vi "HelpMap.vi"(3 "Control ID":string, 4 "Subitem Help ID":string, 5 "Standard Help ID":string) -> (0 "Control Help Description":string, 1 "Subitem Help Info":T1, 2 "Standard Help Info":T1)   [LabVIEW 2017, in "Get DDT Properties.lvlib" / "Get DDT Properties.xnode"]
uses:
  <vilib>/express/express signal manip/GetorSetDDTAttributes/Get DDT attributes/Get DDT Properties.xnode
panel:
  in  "Control Description":string[](array[string])=["Specifies the index of the signal whose attributes you want to retrieve. The default is 0.", "Specifies the dynamic data that contains the input signal or signals.", "Specifies the index of the signal whose attributes you want to retrieve.", "Describes error conditions that occur before this node runs.", "Returns <B>Signals In</B> unchanged.", "Contains error information. This output provides standard error out functionality.", "Returns the name of the signal.", "Returns the time mode of the signal.", "Returns the timestamp of the signal.", "Returns the start timestamp of the signal.", "Returns the X dimension of the signal.", "Returns the unit of measurement of the signal.", "Specifies whether to return the unit of measurement of the signal.", "Specifies whether to return the X dimension of the signal.", "Specifies whether to return the timestamp of the signal.", "Specifies whether to return the time mode of the signal.", "Specifies whether to return the name of the signal.", "Specifies whether to return the start timestamp of the signal."]
  in  "DNL_Control IDs":string[](array[string])=["Signal Index", "Signals In", "Signal Index", "error in", "Signals Out", "error out", "Signal Name", "Time Mode", "Timestamp", "Start Timestamp", "X Dimension", "Unit", "Unit", "X dimension", "Timestamp", "Time mode", "Signal name", "Start timestamp"]
  in  "Subitem Help Clusters":T2(array[cluster])
  in  "DNL_Subitem Help IDs":string[](array[string])
  in  "Standard Help Clusters":T2(array[cluster])=[{"Description"="Retrieves the attributes of the dynamic data you wire to <B>Signals In</B>.", "Path"=path "<helpdir>/lvexpress.chm", "Tag"="get_ddt_attributes.html"}]
  in  "DNL_Standard Help IDs":string[](array[string])=["Default"]
  # "Description"
  # "Path"
  # "Tag"
  # "Description"
  # "Path"
  # "Tag"
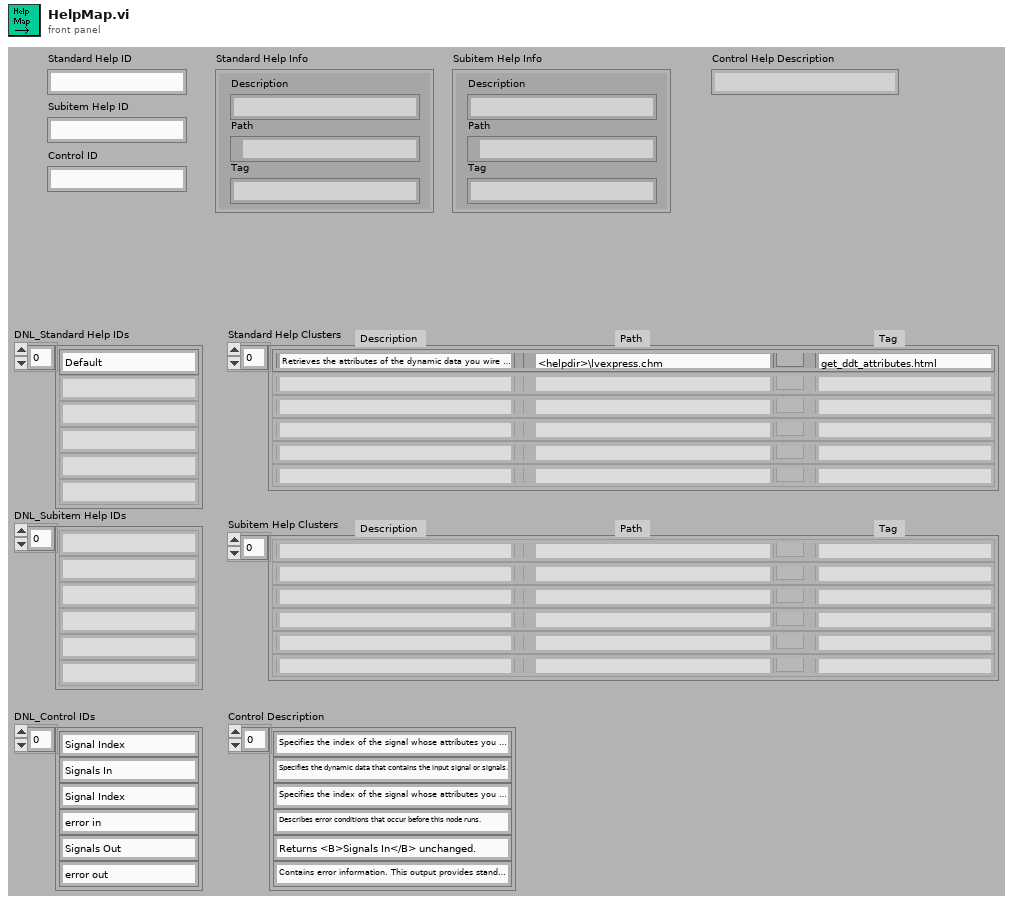
[diagram p1: front panel]
types:
  T1 = cluster{"Description":string, "Path":path, "Tag":string}
  T2 = cluster{"Description":string, "Path":path, "Tag":string}[]
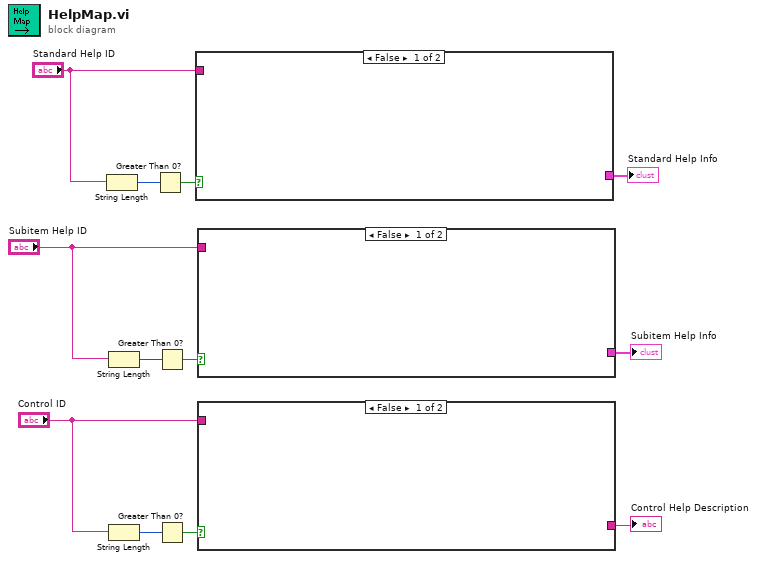
[diagram p0: block diagram]
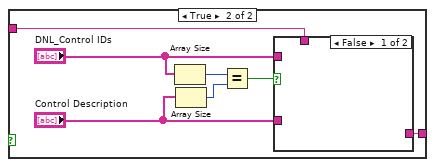
[diagram p2: hidden frame]
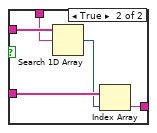
[diagram p3: hidden frame]
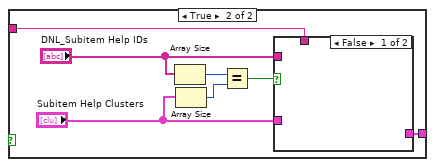
[diagram p4: hidden frame]
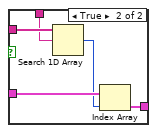
[diagram p5: hidden frame]
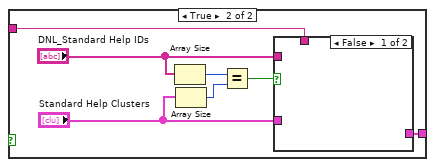
[diagram p6: hidden frame]
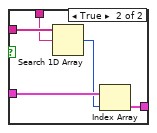
[diagram p7: hidden frame]
diagram:
  n1 = String Length(string="Standard Help ID") -> (length=w12:i32)
  n2 = String Length(string="Subitem Help ID") -> (length=w7:i32)
  n3 = String Length(string="Control ID") -> (length=w4:i32)
  n4 = Greater Than 0?(x=w12) -> (x > 0?=w11:bool)
  n5 = Greater Than 0?(x=w7) -> (x > 0?=w8:bool)
  n6 = Greater Than 0?(x=w4) -> (x > 0?=w3:bool)
  n7 = case shown="False" w11 {
    tunnel: "Standard Help ID" -> [_ w16]
    tunnel: [_ w13] -> w9
    frame False {
    }
    frame True {
      n8 = Array Size(array="DNL_Standard Help IDs") -> (size(s)=w19:i32)
      n9 = Array Size(array="Standard Help Clusters") -> (size(s)=w18:i32)
      n10 = Equal?(x=w19, y=w18) -> (x = y?=w17:bool)
      n11 = case shown="False" w17 {
        tunnel: w16 -> [_ w23]
        tunnel: "DNL_Standard Help IDs" -> [_ w24]
        tunnel: "Standard Help Clusters" -> [_ w22]
        tunnel: [_ w20] -> w13
        frame False {
        }
        frame True {
          n12 = Search 1D Array(1D array=w24, element=w23) -> (index of element=w21:i32)  [unwired: 1 out]
          n13 = Index Array(array=w22, index=w21) -> (element=w20:T1)
        }
      }
    }
  }
  "Standard Help Info" <- w9
  n14 = case shown="False" w8 {
    tunnel: "Subitem Help ID" -> [_ w28]
    tunnel: [_ w27] -> w5
    frame False {
    }
    frame True {
      n15 = Array Size(array="DNL_Subitem Help IDs") -> (size(s)=w31:i32)
      n16 = Array Size(array="Subitem Help Clusters") -> (size(s)=w30:i32)
      n17 = Equal?(x=w31, y=w30) -> (x = y?=w29:bool)
      n18 = case shown="False" w29 {
        tunnel: w28 -> [_ w35]
        tunnel: "DNL_Subitem Help IDs" -> [_ w36]
        tunnel: "Subitem Help Clusters" -> [_ w34]
        tunnel: [_ w32] -> w27
        frame False {
        }
        frame True {
          n19 = Search 1D Array(1D array=w36, element=w35) -> (index of element=w33:i32)  [unwired: 1 out]
          n20 = Index Array(array=w34, index=w33) -> (element=w32:T1)
        }
      }
    }
  }
  "Subitem Help Info" <- w5
  n21 = case shown="False" w3 {
    tunnel: "Control ID" -> [_ w40]
    tunnel: [_ w39] -> w1
    frame False {
    }
    frame True {
      n22 = Array Size(array="DNL_Control IDs") -> (size(s)=w43:i32)
      n23 = Array Size(array="Control Description") -> (size(s)=w42:i32)
      n24 = Equal?(x=w43, y=w42) -> (x = y?=w41:bool)
      n25 = case shown="False" w41 {
        tunnel: w40 -> [_ w47]
        tunnel: "DNL_Control IDs" -> [_ w48]
        tunnel: "Control Description" -> [_ w46]
        tunnel: [_ w44] -> w39
        frame False {
        }
        frame True {
          n26 = Search 1D Array(1D array=w48, element=w47) -> (index of element=w45:i32)  [unwired: 1 out]
          n27 = Index Array(array=w46, index=w45) -> (element=w44:string)
        }
      }
    }
  }
  "Control Help Description" <- w1
